vi "Remove Target from Path.vi"(8 "error in (no error)":errorcluster, 11 "NodePath":string) -> (0 "error out":errorcluster, 3 "PathArrayToString":string)   [LabVIEW 2023, in "Instrument Addon Scripting API.lvlib"]
uses:
  Instrument Addon Scripting API.lvlib
  NationalInstruments.VeriStand
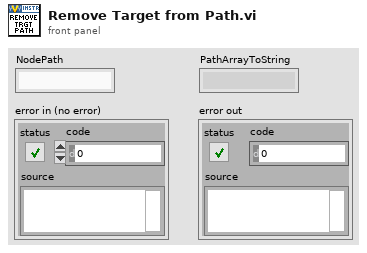
[diagram p1: front panel]
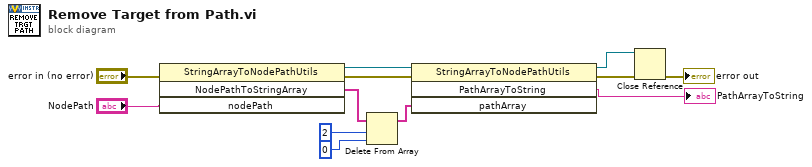
[diagram p0: block diagram]
diagram:
  n1 = invoke class="StringArrayToNodePathUtils" method="NodePathToStringArray"(error in="error in (no error)", "nodePath"="NodePath") -> (reference out=w12:refnum<k24>, error out=w10:errorcluster, "NodePathToStringArray"=w4:string[])  [unwired: 2 in, 1 out]
  n2 = Delete From Array(array=w4, length=2, index=0) -> (array with subset deleted=w9:string[])  [unwired: 1 out]
  n3 = invoke class="StringArrayToNodePathUtils" method="PathArrayToString"(reference=w12, error in=w10, "pathArray"=w9) -> (reference out=w2:refnum<k24>, error out=w3:errorcluster, "PathArrayToString"=→"PathArrayToString":string)  [unwired: 1 in, 1 out]
  n4 = Close Reference(reference=w2, error in (no error)=w3) -> (error out=→"error out":errorcluster)
